vi "Array-Last Value.vi"(1 "array":dbl[](array[numeric])) -> (0 "element":dbl)   [LabVIEW 2020]
panel:
  # "Extracts the last element of an array"
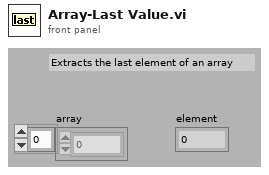
[diagram p1: front panel]
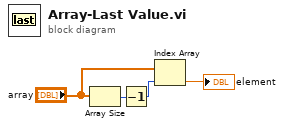
[diagram p0: block diagram]
diagram:
  n1 = Array Size(array="array") -> (size(s)=w4:i32)
  n2 = Decrement(x=w4) -> (x-1=w3:i32)
  n3 = Index Array(array="array", index=w3) -> (element=→"element":dbl)
